vi "RFM Control and Status.Local CSR.Status LED.Set.vi"(8 "error in (no error)":errorcluster, 10 "Status LED State":bool, 11 "GE 5565PIORC":refnum<class "GE 5565PIORC.lvclass">) -> (0 "error out":errorcluster, 3 "GE 5565PIORC out":refnum<class "GE 5565PIORC.lvclass">)   [LabVIEW 2016, in "GE 5565PIORC.lvclass"]
uses:
  GE 5565PIORC.lvclass
  Controls/Registers.RFM Control and Status.ctl
  GE 5565PIORC.lvclass/GE 5565PIORC.ctl
  <vilib>/Instr/_visa.llb/VISA Register Access Address Space.ctl
  Binary Operations/Set Bits U32.vi
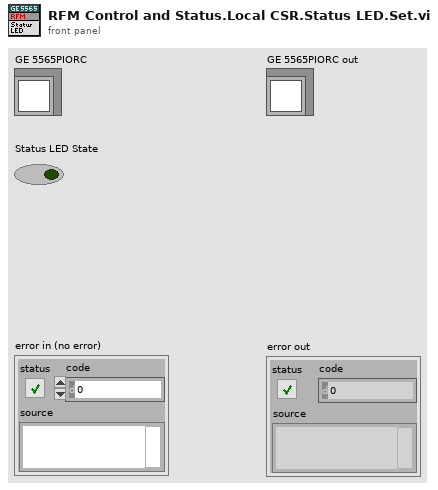
[diagram p1: front panel]
types:
  T1 = typedef "GE 5565PIORC.lvclass/Registers.RFM Control and Status.ctl" = enum16{"Board Revision", "Board ID", "Board Revision Build", "Node ID", "Local Control and Status", "Local Interrupt Status", "Local Interrupt Enable", "Network Target Data", "Network Target Node", "Network Interrupt Command", "Interrupt 1 Sender Data", "Interrupt 1 Sender ID", "Interrupt 2 Sender Data", "Interrupt 2 Sender ID", "Interrupt 3 Sender Data", "Interrupt 3 Sender ID", "Interrupt 4 Sender Data", "Interrupt 4 Sender ID"}
  T2 = typedef "VISA Register Access Address Space.ctl" = u16
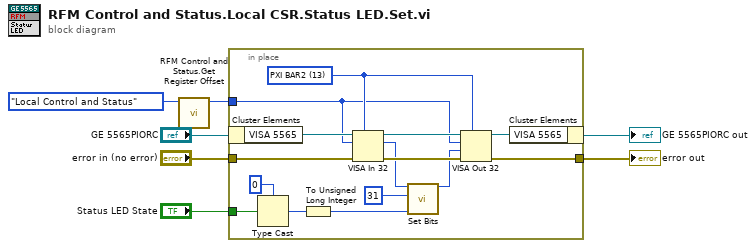
[diagram p0: block diagram]
diagram:
  n1 = call "RFM Control and Status.Get Register Offset.vi"("RFM Control and Status Register"=Registers.RFM_Control_and_Status."Local Control and Status") -> ("Offset"=w1:u32)  [unwired: 10 in]
  n2 = in-place {
    in-place-border: "error in (no error)" -> [w21]
    in-place-border: [w17] -> w5
    in-place-border: "Status LED State" -> [w12]
    in-place-border: w1 -> [w8]
    w14 = T2 13 items=["VXI/VME A16"=1, "VXI/VME A24"=2, "VXI/VME A32"=3, "VXI/VME A64"=4, "PXI Memory Allocations"=9, "PXI Configuration"=10, "PXI BAR0"=11, "PXI BAR1"=12, "PXI BAR2"=13, "PXI BAR3"=14, "PXI BAR4"=15, "PXI BAR5"=16] ("Address Space")
    n3 = in-place-cluster #1("GE 5565PIORC") -> ("VISA 5565"=w22:refnum<visa-resource-name>)
    n4 = Type Cast(type=u8 0, x=w12) -> (*(type *) &x=w10:u8)
    n5 = To Unsigned Long Integer(number=w10) -> (unsigned 32bit integer=w9:u32)
    n6 = VISA In 32(7:w14, 8:w21, 10:w8, 11:w22) -> (0:w19:errorcluster, 2:w15:u32, 3:w20:refnum<visa-resource-name>)
    n7 = call-poly "Set Bits.vi"("Value (0)"=w9, "Start Index (0)"=u8 31, "Register in"=w15) -> ("Register out"=w16:u32)  [unwired: 6 in, 2 out]
    n8 = VISA Out 32(7:w14, 8:w19, 9:w16, 10:w8, 11:w20) -> (0:w17:errorcluster, 3:w18:refnum<visa-resource-name>)
    n9 = in-place-cluster #1("VISA 5565"=w18) -> (→"GE 5565PIORC out":refnum<class "GE 5565PIORC.lvclass">)
  }
  "error out" <- w5
